vi "positionCalc.vi"(6 "Velocity Timeout (s)":dbl=1.0 format="%#_13g", 9 "Right Now":timestamp, 10 "Distance per Stripe (m)":dbl, 11 "Laser":T2) -> (3 "Position Data":T1)   [LabVIEW 2017]
uses:
  Type Defs/laserReading.ctl
  Type Defs/positionData.ctl
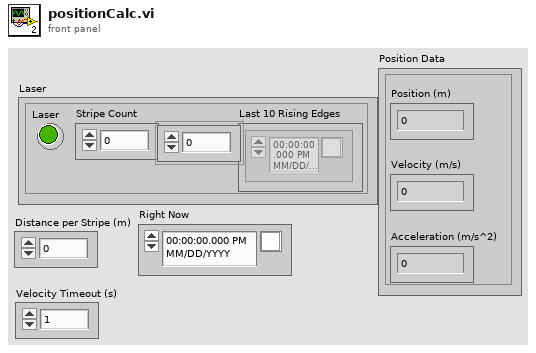
[diagram p1: front panel]
types:
  T1 = typedef "positionData.ctl" = cluster{"Position (m)":dbl, "Velocity (m/s)":dbl, "Acceleration (m/s^2)":dbl}
  T2 = typedef "laserReading.ctl" = cluster{"Laser":bool, "Stripe Count":u32, "Last 10 Rising Edges":timestamp[]}
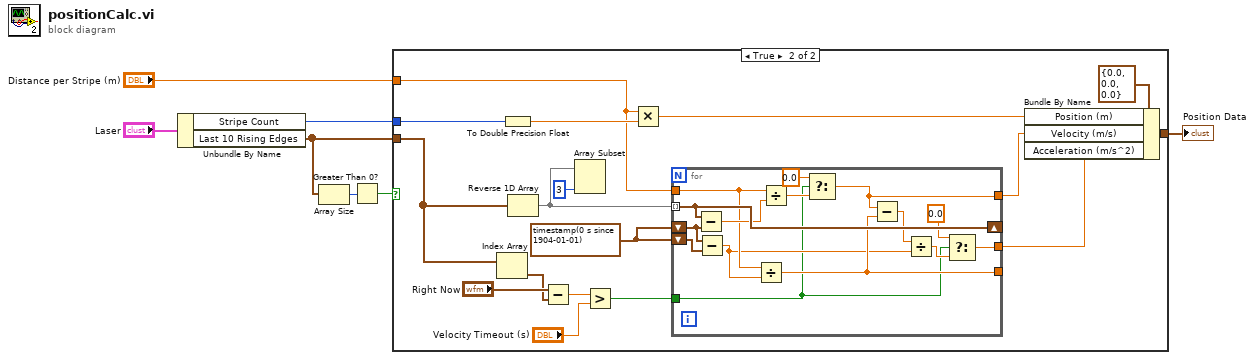
[diagram p0: block diagram]
diagram:
  n1 = Unbundle By Name("Laser") -> ("Stripe Count"=w6:u32, "Last 10 Rising Edges"=w3:timestamp[])
  n2 = Array Size(array=w3) -> (size(s)=w2:i32)
  n3 = Greater Than 0?(x=w2) -> (x > 0?=w1:bool)
  n4 = case shown="True" w1 {
    tunnel: w6 -> [_ w24]
    tunnel: [_ w21] -> w5
    tunnel: "Distance per Stripe (m)" -> [_ w19]
    tunnel: w3 -> [_ w8]
    frame False {
    }
    frame True {
      w16 = timestamp(0 s since 1904-01-01) ("Time Stamp")
      n5 = Index Array(array=w8) -> (element=w12:timestamp)  [unwired: 1 in]
      n6 = To Double Precision Float(number=w24) -> (double precision float=w23:dbl)
      n7 = Reverse 1D Array(array=w8) -> (reversed array=w15:timestamp[])
      n8 = Subtract(x="Right Now", y=w12) -> (x-y=w11:dbl)
      n9 = Array Subset(array=w15, length=3) -> ()  [unwired: 1 in, 1 out]
      n10 = Greater?(x=w11, y="Velocity Timeout (s)") -> (0:w9:bool)
      n11 = Multiply(x=w19, y=w23) -> (x*y=w20:dbl)
      n12 = for {
        tunnel: w15 -> [w39] mode=indexing
        tunnel: w19 -> [w35]
        shift-right: [w39] -> _
        shift-left: w16 -> [w38]
        shift-left: w16 -> [w37]
        tunnel: [w29] -> w18
        tunnel: [w34] -> _
        tunnel: [w25] -> w17
        tunnel: w9 -> [w27]
        n13 = Subtract(x=w39, y=w38) -> (x-y=w36:dbl)
        n14 = Subtract(x=w38, y=w37) -> (x-y=w32:dbl)
        n15 = Divide(x=w35, y=w32) -> (x/y=w34:dbl)
        n16 = Divide(x=w35, y=w36) -> (x/y=w31:dbl)
        n17 = Select(t=0.0, s=w27, f=w31) -> (s? t:f=w29:dbl)
        n18 = Subtract(x=w29, y=w34) -> (x-y=w33:dbl)
        n19 = Divide(x=w33, y=w32) -> (x/y=w28:dbl)
        n20 = Select(t=0.0, s=w27, f=w28) -> (s? t:f=w25:dbl)
      }
      n21 = Bundle By Name(cluster=T1 {"Position (m)"=0.0, "Velocity (m/s)"=0.0, "Acceleration (m/s^2)"=0.0} ("Position Data"), "Position (m)"=w20, "Velocity (m/s)"=w18, "Acceleration (m/s^2)"=w17) -> (w21:T1)
    }
  }
  "Position Data" <- w5
